vi "CRYGet Graph Data in Rename.vi"(8 "New Name":string, 9 "Old Name":string, 10 "Graph VI Ref":refnum<vi>) -> (2 "Visible Rows":i32[](array[numeric]))   [LabVIEW 2013]
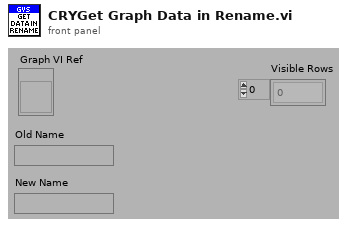
[diagram p1: front panel]
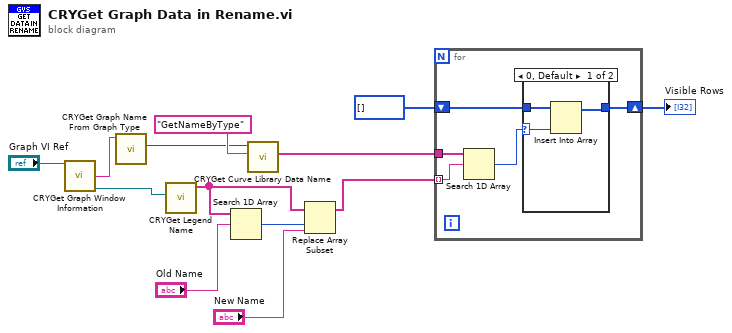
[diagram p0: block diagram]
diagram:
  n1 = call "CRYGet Graph Window Information.vi"("pGraph VI In"="Graph VI Ref") -> ("Graph Type Out"=w2:string, "Legend Ref Out"=w3:refnum<vi>)  [unwired: 4 in, 9 out]
  n2 = call "CRYGet Graph Name From Graph Type.vi"("Graph Type"=w2) -> ("Type"=w1:enum16{"Curves", "Values", "Results", "WFM"})  [unwired: 9 in, 1 out]
  n3 = call "CRYGet Legend Name.vi"("MCListbox Refnum"=w3) -> ("Names Out"=w9:string[])  [unwired: 2 in, 8 out]
  n4 = Search 1D Array(1D array=w9, element="Old Name") -> (index of element=w8:i32)  [unwired: 1 out]
  n5 = call "CRYGet Curve Library Data Name.vi"("sAction"="GetNameByType", "Type"=w1) -> ("sNames"=w11:string[])  [unwired: 4 in, 5 out]
  n6 = Replace Array Subset(array=w9, new element="New Name", index=w8) -> (w6:string[])
  n7 = for {
    tunnel: w6 -> [w17] mode=indexing
    tunnel: w11 -> [w18]
    shift-right: [w14] -> w12
    shift-left: i32[] [] -> [w15]
    n8 = Search 1D Array(1D array=w18, element=w17) -> (index of element=w16:i32)  [unwired: 1 in]
    n9 = case shown="0, Default" w16 {
      selector: w16 -> [w21 _]
      tunnel: [w19 w22] -> w14
      tunnel: w15 -> [w20 w22]
      frame 0, Default {
        n10 = Insert Into Array(array=w20, new element=w21) -> (w19:i32[])  [unwired: 1 in]
      }
      frame -1 {
      }
    }
  }
  "Visible Rows" <- w12
